vi "SetCtrlPropGenPol.vi"   [LabVIEW 2010]
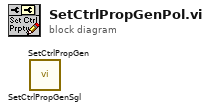
[diagram p0: block diagram]
diagram:
  n1 = call <userlib>:"SetCtrlPropGenSgl.vi"() -> ()  [unwired: 6 in, 2 out]
  n2 = call <userlib>:"SetCtrlPropGen.vi"() -> ()  [unwired: 6 in, 2 out]
